vi "MCL Correct Driver Version.vi"() -> (3 "function return":bool)   [LabVIEW 2017, in "Madlib.lvlib"]
doc: "MADLIB_API bool MCL_CorrectDriverVersion();"
uses:
  Madlib.lvlib
  Madlib.dll
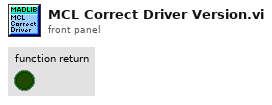
[diagram p1: front panel]
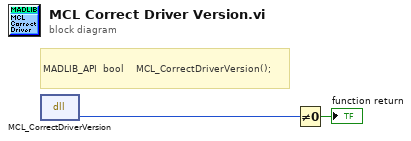
[diagram p0: block diagram]
diagram:
  # "MADLIB_API  bool    MCL_CorrectDriverVersion();"
  n1 = dll-call lib="C:/Users/francesco/dev/pump-probe/Piezo/lvlib/Madlib.*" fn="MCL_CorrectDriverVersion"() -> (w1:u8)  [unwired: 3 in, 2 out]
  n2 = Not Equal To 0?(x=w1) -> (x != 0?=→"function return":bool)
